vi "Housekeeping.vi"(8 "error in (no error)":errorcluster, 11 "CIFTemplatePlugin in":refnum<class "TemplatePlugin.lvclass">) -> (0 "error out":errorcluster, 3 "CIFTemplatePlugin out":refnum<class "TemplatePlugin.lvclass">)   [LabVIEW 2021, in "TemplatePlugin.lvclass"]
uses:
  TemplatePlugin.lvclass
  TemplatePlugin.lvclass/TemplatePlugin.ctl
  CIF-LVCore/src/CIFCore/Class/CIFCorePlugin.lvclass
  CIF-LVCore/src/CIFCore/Class/Typedef/Energized States.ctl
  D:/dev/CIF-LVCore/src/CIFCore/Class/CIFCorePlugin.lvclass
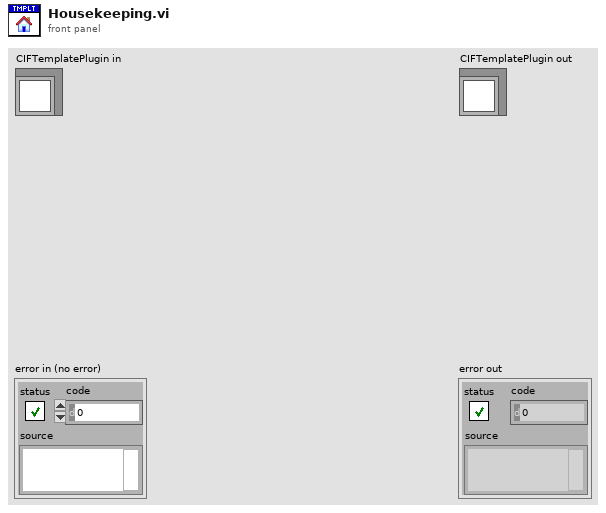
[diagram p1: front panel]
types:
  T1 = typedef "CIFCorePlugin.lvclass/Energized States.ctl" = enum16{"Listen", "Prepare", "Execute", "Housekeep", "Cleanup", "Destroy"}
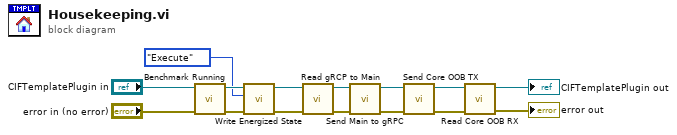
[diagram p0: block diagram]
diagram:
  n1 = call "Benchmark Running.vi"("error in (no error)"="error in (no error)", "CIFCorePlugin in"="CIFTemplatePlugin in") -> ("error out"=w6:errorcluster, "CIFCorePlugin out"=w14:refnum<class "TemplatePlugin.lvclass">)  [unwired: 8 in]
  n2 = call "Write Energized State.vi"("error in (no error)"=w6, "Energized State"=Energized_States."Execute", "CIFCorePlugin in"=w14) -> ("error out"=w10:errorcluster, "CIFCorePlugin out"=w12:refnum<class "TemplatePlugin.lvclass">)  [unwired: 7 in]
  n3 = call "Read gRCP to Main.vi"("error in (no error)"=w10, "CIFTemplatePlugin in"=w12) -> ("error out"=w2:errorcluster, "CIFTemplatePlugin out"=w1:refnum<class "TemplatePlugin.lvclass">)  [unwired: 8 in]
  n4 = call "Send Main to gRPC.vi"("error in (no error)"=w2, "CIFTemplatePlugin in"=w1) -> ("error out"=w5:errorcluster, "CIFTemplatePlugin out"=w11:refnum<class "TemplatePlugin.lvclass">)  [unwired: 8 in]
  n5 = call "Send Core OOB TX.vi"("error in (no error)"=w5, "CIFCorePlugin in"=w11) -> ("error out"=w3:errorcluster, "CIFCorePlugin out"=w15:refnum<class "TemplatePlugin.lvclass">)  [unwired: 8 in]
  n6 = call "Read Core OOB RX.vi"("error in (no error)"=w3, "CIFCorePlugin in"=w15) -> ("error out"=→"error out":errorcluster, "CIFCorePlugin out"=→"CIFTemplatePlugin out":refnum<class "TemplatePlugin.lvclass">)  [unwired: 8 in]
